vi "Test InterCircles.vi"() -> ()   [LabVIEW 2013]
panel:
  out "2D Picture":picture
  in  "r 1":dbl
  in  "r 0":dbl
  out "exist":bool
  in  "c 1":dbl[](array[numeric])
  in  "c 0":dbl[](array[numeric])
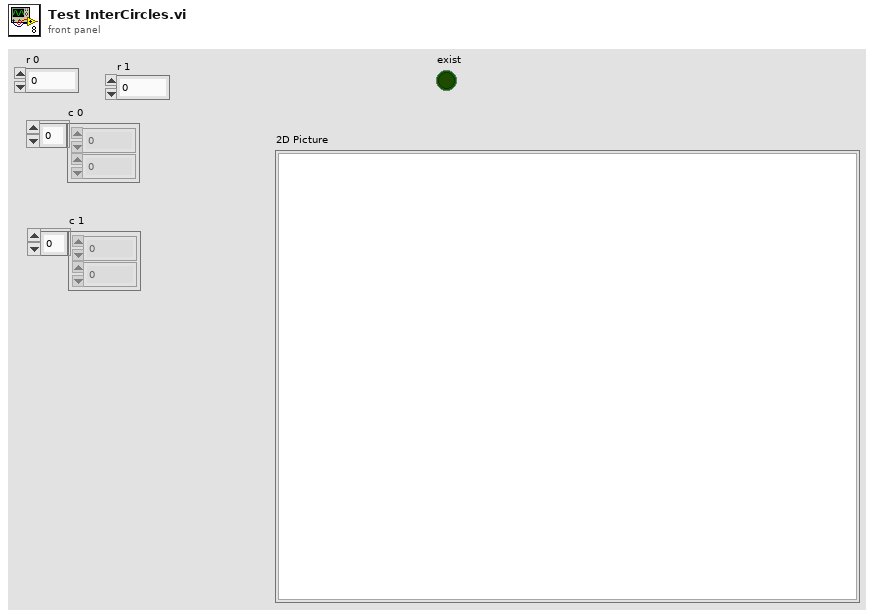
[diagram p1: front panel]
types:
  T1 = cluster{"Width":u16, "Style":enum32{"Solid", "Dash", "Dot", "DashDot", "DashDotDot"}}
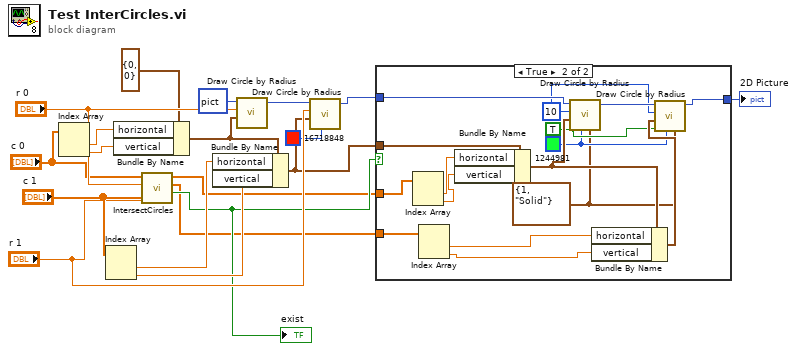
[diagram p0: block diagram]
diagram:
  n1 = Index Array(array="c 0") -> (element #1=w16:dbl, element #2=w15:dbl)  [unwired: 2 in]
  n2 = Index Array(array="c 1") -> (element #1=w11:dbl, element #2=w10:dbl)  [unwired: 2 in]
  n3 = Bundle By Name(cluster=cluster{"horizontal":i16, "vertical":i16} {"horizontal"=0, "vertical"=0} ("pixel center"), "horizontal"=w16, "vertical"=w15) -> (w13:cluster{"horizontal":i16, "vertical":i16})
  n4 = call "IntersectCircles.vi"("r 1"="r 1", "c 1"="c 1", "r 0"="r 0", "c 0"="c 0") -> ("exist"=w6:bool, "p 1"=w2:dbl[], "p 0"=w4:dbl[])  [unwired: 5 in]
  "exist" <- w6
  n5 = Bundle By Name(cluster=w13, "horizontal"=w11, "vertical"=w10) -> (w5:cluster{"horizontal":i16, "vertical":i16})
  n6 = call <vilib>:"Draw Circle by Radius.vi"("pixel center"=w13, "radius"="r 0", "picture"=picture data[5B]) -> ("new picture"=w8:picture)  [unwired: 8 in]
  n7 = call <vilib>:"Draw Circle by Radius.vi"("color(black)"=u32 16718848, "pixel center"=w5, "radius"="r 1", "picture"=w8) -> ("new picture"=w3:picture)  [unwired: 7 in]
  n8 = case shown="True" w6 {
    tunnel: w5 -> [_ w36]
    tunnel: w4 -> [_ w35]
    tunnel: w3 -> [w20 w32]
    tunnel: w2 -> [_ w28]
    tunnel: [w20 w21] -> w1
    frame False {
    }
    frame True {
      w22 = T1 {"Width"=1, "Style"=enum."Solid"} ("pen")
      w23 = u32 1244981 ("color(black)")
      w24 = TRUE ("fill?(F)")
      w30 = i16 10 ("radius")
      n9 = Index Array(array=w35) -> (element #1=w34:dbl, element #2=w33:dbl)  [unwired: 2 in]
      n10 = Index Array(array=w28) -> (element #1=w27:dbl, element #2=w26:dbl)  [unwired: 2 in]
      n11 = Bundle By Name(cluster=w36, "horizontal"=w34, "vertical"=w33) -> (w29:cluster{"horizontal":i16, "vertical":i16})
      n12 = call <vilib>:"Draw Circle by Radius.vi"("pen"=w22, "color(black)"=w23, "fill?(F)"=w24, "pixel center"=w29, "radius"=w30, "picture"=w32) -> ("new picture"=w31:picture)  [unwired: 5 in]
      n13 = Bundle By Name(cluster=w29, "horizontal"=w27, "vertical"=w26) -> (w25:cluster{"horizontal":i16, "vertical":i16})
      n14 = call <vilib>:"Draw Circle by Radius.vi"("pen"=w22, "color(black)"=w23, "fill?(F)"=w24, "pixel center"=w25, "radius"=w30, "picture"=w31) -> ("new picture"=w21:picture)  [unwired: 5 in]
    }
  }
  "2D Picture" <- w1
